vi "Start Remote Node.vi"(8 "Error In":errorcluster, 10 "Node-ID":u8, 11 "ICommunicate":refnum<class "ICommunicate.lvclass">) -> (0 "Error Out":errorcluster)   [LabVIEW 2024, in "CANopen Master.lvlib" / "Network Mangement.lvclass"]
doc: "The NMT master uses the NMT service start remote node to change the NMT state of the selected \nNMT slaves. The new NMT state shall be the NMT state operational."
uses:
  Network Mangement.lvclass
  Network Mangement.lvclass/Network Mangement.ctl
  CANopen Message/CANopen Message.lvclass
  HAL/Source/Interfaces/ICommunicate/ICommunicate.lvclass
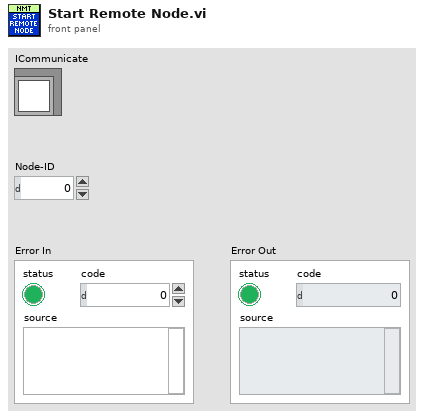
[diagram p1: front panel]
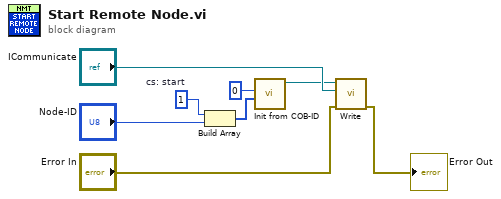
[diagram p0: block diagram]
diagram:
  w2 = u8 1  # cs: start
  n1 = Build Array(w2, "Node-ID") -> (w1:u8[])
  n2 = call "Init from COB-ID.vi"("Data"=w1, "COB-ID"=u32 0) -> ("CANopen Message out"=w6:refnum<class "CANopen Message.lvclass">)  [unwired: 9 in]
  n3 = call "Write.vi"("error in"="Error In", "ICommunicate"="ICommunicate", "CANopen Message in"=w6) -> ("error out"=→"Error Out":errorcluster)  [unwired: 7 in, 1 out]
